vi "verify setup parameters.vi"(8 "error in (no error)":errorcluster, 11 "Channel in":refnum<class "Channel.lvclass">) -> (0 "error out":errorcluster, 3 "Channel out":refnum<class "Channel.lvclass">)   [LabVIEW 2018, in "Channel.lvclass"]
uses:
  Channel.lvclass
  Channel.lvclass/Channel.ctl
  Simulated_CCD_Camera/Simulated_CCD_Camera.lvclass/Simulated_CCD_Camera.ctl
  Simulated_CCD_Camera/Simulated_CCD_Camera.lvclass
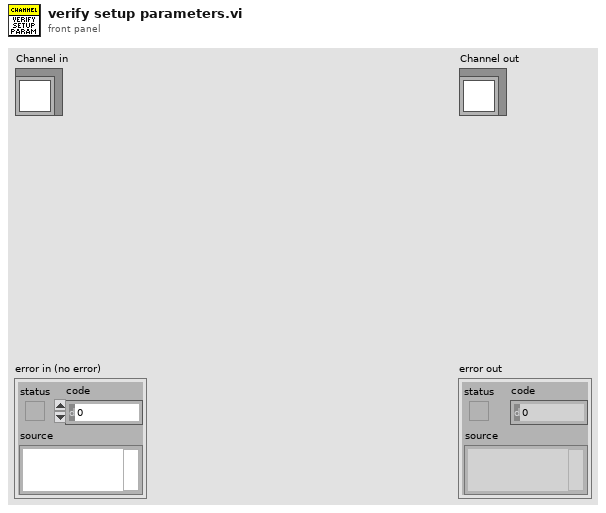
[diagram p1: front panel]
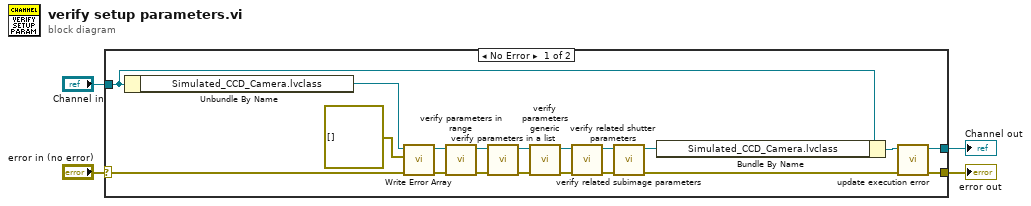
[diagram p0: block diagram]
diagram:
  n1 = case shown="No Error" "error in (no error)" {
    selector: "error in (no error)" -> [w12 w25]
    tunnel: [w6 w25] -> w3
    tunnel: [w7 w24] -> w1
    tunnel: "Channel in" -> [w23 w24]
    frame No Error {
      n2 = Unbundle By Name(w23) -> ("Simulated_CCD_Camera.lvclass"=w11:refnum<class "Simulated_CCD_Camera.lvclass">)
      n3 = call "Write Error Array.vi"("error in (no error)"=w12, "Errors array"=errorcluster[] [], "Simulated_CCD_Camera in"=w11) -> ("error out"=w13:errorcluster, "Simulated_CCD_Camera out"=w14:refnum<class "Simulated_CCD_Camera.lvclass">)  [unwired: 7 in]
      n4 = call "verify parameters in range.vi"("error in (no error)"=w13, "Simulated_CCD_Camera in"=w14) -> ("error out"=w22:errorcluster, "Simulated_CCD_Camera out"=w21:refnum<class "Simulated_CCD_Camera.lvclass">)  [unwired: 8 in]
      n5 = call "verify parameters in a list.vi"("error in (no error)"=w22, "Simulated_CCD_Camera in"=w21) -> ("error out"=w15:errorcluster, "Simulated_CCD_Camera out"=w16:refnum<class "Simulated_CCD_Camera.lvclass">)  [unwired: 8 in]
      n6 = call "verify parameters generic.vi"("error in (no error)"=w15, "Simulated_CCD_Camera in"=w16) -> ("error out"=w17:errorcluster, "Simulated_CCD_Camera out"=w18:refnum<class "Simulated_CCD_Camera.lvclass">)  [unwired: 8 in]
      n7 = call "verify related shutter parameters.vi"("error in (no error)"=w17, "Simulated_CCD_Camera in"=w18) -> ("error out"=w19:errorcluster, "Simulated_CCD_Camera out"=w20:refnum<class "Simulated_CCD_Camera.lvclass">)  [unwired: 8 in]
      n8 = call "verify related subimage parameters.vi"("error in (no error)"=w19, "Simulated_CCD_Camera in"=w20) -> ("error out"=w5:errorcluster, "Simulated_CCD_Camera out"=w9:refnum<class "Simulated_CCD_Camera.lvclass">)  [unwired: 8 in]
      n9 = Bundle By Name(cluster=w23, "Simulated_CCD_Camera.lvclass"=w9) -> (w8:refnum<class "Channel.lvclass">)
      n10 = call "update execution error.vi"("error in (no error)"=w5, "Channel in"=w8) -> ("error out"=w6:errorcluster, "Channel out"=w7:refnum<class "Channel.lvclass">)  [unwired: 8 in]
    }
    frame Error {
    }
  }
  "error out" <- w3
  "Channel out" <- w1
